vi "DPO4034 Save Recall Setup.vi"(8 "error in (no error)":errorcluster, 9 "Save/Recall":u16(ring) items=["Save", "Recall"], 10 "Location":u16(ring)=1 items=["Location 1"=1, "Location 2"=2, "Location 3"=3, "Location 4"=4, "Location 5"=5, "Location 6"=6, "Location 7"=7, "Location 8"=8, "Location 9"=9, "Location 10"=10], 11 "VISA resource name":refnum<visa-resource-name>) -> (0 "error out":errorcluster, 3 "VISA resource name out":refnum<visa-resource-name>)   [LabVIEW 2012]
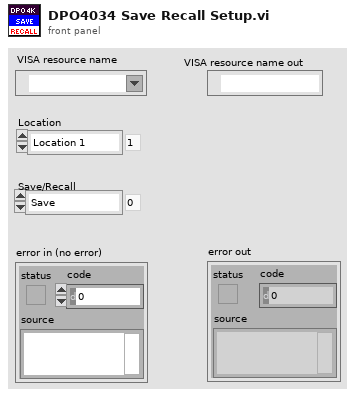
[diagram p1: front panel]
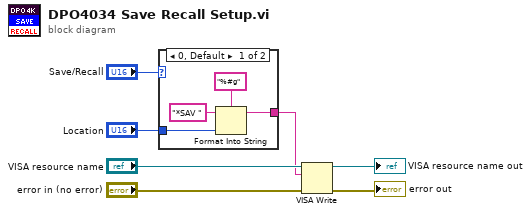
[diagram p0: block diagram]
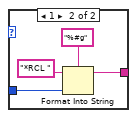
[diagram p2: hidden frame]
diagram:
  n1 = case shown="0, Default" "Save/Recall" {
    tunnel: "Location" -> [w11 w13]
    tunnel: [w8 w12] -> w5
    frame 0, Default {
      n2 = Format Into String(format string="%#g", initial string="*SAV ", w11) -> (resulting string=w8:string)  [unwired: 1 in, 1 out]
    }
    frame 1 {
      n3 = Format Into String(format string="%#g", initial string="*RCL ", w13) -> (resulting string=w12:string)  [unwired: 1 in, 1 out]
    }
  }
  n4 = VISA Write(VISA resource name="VISA resource name", write buffer=w5, error in (no error)="error in (no error)") -> (VISA resource name out=→"VISA resource name out":refnum<visa-resource-name>, error out=→"error out":errorcluster)  [unwired: 1 out]
